vi "Create Parameters List.vi"(11 "ctl label -> value var[]":map{string, variant[]}(c390)) -> (3 "Set of ctl label -> value var combos":set{map{string, variant}}(c389))   [LabVIEW 2020, in "Approval Tests.lvlib"]
uses:
  Approval Tests.lvlib
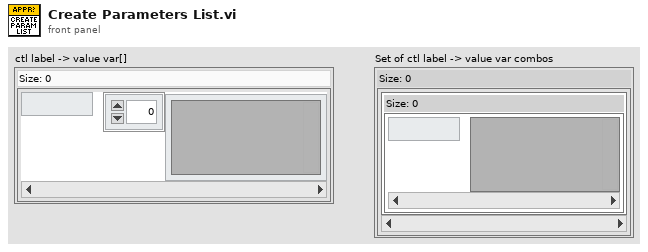
[diagram p1: front panel]
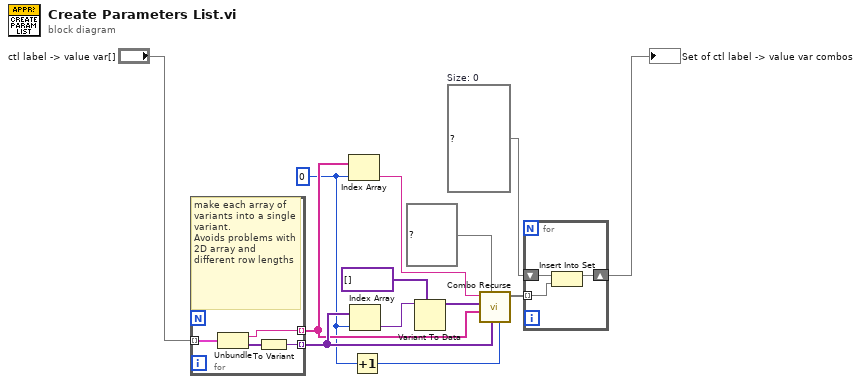
[diagram p0: block diagram]
diagram:
  w1 = set{map{string, variant}} {}  # Size: 0
  w4 = 0 ("index")
  n1 = for {
    tunnel: "ctl label -> value var[]" -> [w17] mode=indexing
    tunnel: [w15] -> w7 mode=indexing
    tunnel: [w14] -> w6 mode=indexing
    # "make each array of variants into a single variant.\nAvoids problems with 2D array and different row lengths"
    n2 = Unbundle(w17) -> ("key"=w14:string, "Array out"=w16:variant[])
    n3 = To Variant(anything=w16) -> (Variant=w15:variant)
  }
  n4 = Index Array(array=w6, index=w4) -> (element=w5:string)
  n5 = Index Array(array=w7, index=w4) -> (element=w8:variant)
  n6 = Increment(x=w4) -> (x+1=w3:i32)
  n7 = Variant To Data(type=variant[] [], Variant=w8) -> (data=w2:variant[])  [unwired: 1 in, 1 out]
  n8 = call "Combo Recurse.vi"("Level"=w3, "All Values"=w7, "Map In"=map{string, variant} {} ("map out"), "All Inputs"=w6, "To Add"=w2, "key"=w5) -> ("Maps Out"=w11:map{string, variant}[])  [unwired: 5 in]
  n9 = for {
    tunnel: w11 -> [w20] mode=indexing
    shift-right: [w19] -> w12
    shift-left: w1 -> [w18]
    n10 = Insert Into Set(10:w20, 11:w18) -> (3:w19:set{map{string, variant}})  [unwired: 1 out]
  }
  "Set of ctl label -> value var combos" <- w12
